vi "reset_start_time.vi"(11 "Mission in":refnum<class "Mission.lvclass">) -> (3 "Mission out":refnum<class "Mission.lvclass">)   [LabVIEW 2011, in "Mission.lvclass"]
uses:
  Mission.lvclass
  Mission.lvclass/Mission.ctl
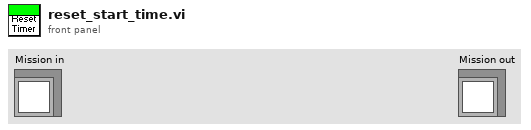
[diagram p1: front panel]
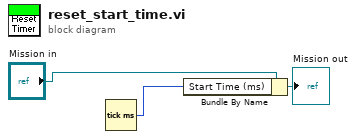
[diagram p0: block diagram]
diagram:
  n1 = Tick Count (ms)() -> (millisecond timer value=w1:u32)
  n2 = Bundle By Name(cluster="Mission in", "Start Time (ms)"=w1) -> (→"Mission out":refnum<class "Mission.lvclass">)
